vi "PWM_Lenkung.vi"(0 "vorne rechts":dbl, 1 "vorne links":dbl, 4 "Schräg links":dbl, 5 "PID Lenkung":T1={"proportional gain (Kc)"=0.71, "integral time (Ti, min)"=2.0, "derivative time (Td, min)"=0.002} {"derivative time (Td, min)" format="%.3f"; "integral time (Ti, min)" format="%.3f"; "proportional gain (Kc)" format="%.3f"}) -> (14 "PWM Lenkung":dbl)   [LabVIEW 2016]
doc: "PID Regelung für Servowert\n05.04.17_Tloe"
uses:
  <vilib>/addons/control/pid/pid.llb/PID (DBL).vi
  <vilib>/addons/control/pid/NI_PID_pid.lvlib
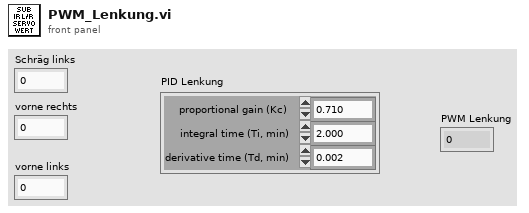
[diagram p1: front panel]
types:
  T1 = cluster{"proportional gain (Kc)":dbl, "integral time (Ti, min)":dbl, "derivative time (Td, min)":dbl}
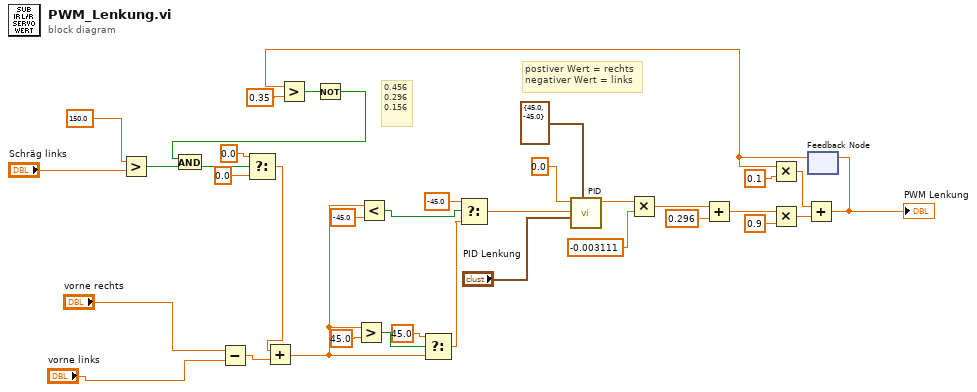
[diagram p0: block diagram]
diagram:
  # "0.456\n0.296\n0.156"
  # "postiver Wert = rechts\nnegativer Wert = links"
  n1 = Greater?(x=150.0 ("y"), y="Schräg links") -> (0:w14:bool)
  n2 = Subtract(x="vorne rechts", y="vorne links") -> (x-y=w11:dbl)
  n3 = feedback #1() -> (w8:dbl)  [unwired: 1 in]
  n4 = Greater?(x=w8, y=0.35) -> (0:w5:bool)
  n5 = Not(x=w5) -> (.not. x?=w4:bool)
  n6 = And(x=w4, y=w14) -> (x .and. y?=w6:bool)
  n7 = Select(t=0.0, s=w6, f=0.0) -> (s? t:f=w9:dbl)
  n8 = Add(x=w9, y=w11) -> (x+y=w12:dbl)
  n9 = Greater?(x=w12, y=45.0) -> (0:w29:bool)
  n10 = Less?(x=w12, y=-45.0) -> (x < y?=w34:bool)
  n11 = Select(t=45.0, s=w29, f=w12) -> (s? t:f=w35:dbl)
  n12 = Select(t=-45.0, s=w34, f=w35) -> (s? t:f=w36:dbl)
  n13 = call-poly <vilib>:"PID.vi"("output range"=cluster{"output high":dbl, "output low":dbl} {"output high"=45.0, "output low"=-45.0}, "PID gains"="PID Lenkung", "process variable"=w36, "setpoint"=0.0) -> ("output"=w28:dbl)  [unwired: 6 in, 1 out]
  n14 = Multiply(x=w28, y=-0.003111) -> (x*y=w24:dbl)
  n15 = Add(x=w24, y=0.296) -> (x+y=w26:dbl)
  n16 = Multiply(x=w8, y=0.1) -> (x*y=w20:dbl)
  n17 = Multiply(x=w26, y=0.9) -> (x*y=w21:dbl)
  n18 = Add(x=w20, y=w21) -> (x+y=w16:dbl)
  "PWM Lenkung" <- w16
  n19 = feedback-in #1(w16) -> ()
